vi "Math-NaN Stats.vi"(7 "Array":dbl[](array[numeric])) -> (4 "NaN Mean":dbl, 6 "NaN SD":dbl, 15 "N":i16)   [LabVIEW 2020]
uses:
  <vilib>/Analysis/NI_AALBase.lvlib
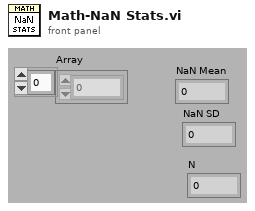
[diagram p1: front panel]
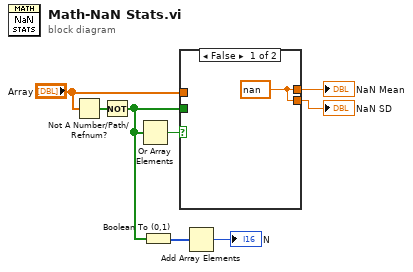
[diagram p0: block diagram]
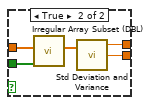
[diagram p2: hidden frame]
diagram:
  n1 = Not A Number/Path/Refnum?(number/path/refnum="Array") -> (NaN/Path/Refnum?=w6:bool[])
  n2 = Not(x=w6) -> (.not. x?=w4:bool[])
  n3 = Or Array Elements(Boolean array=w4) -> (logical OR=w5:bool)
  n4 = Boolean To (0,1)(Boolean=w4) -> (0, 1=w3:i16[])
  n5 = case shown="False" w5 {
    tunnel: [w9 w11] -> w8
    tunnel: "Array" -> [_ w14]
    tunnel: w4 -> [_ w13]
    tunnel: [w9 w10] -> w1
    frame False {
      w9 = nan ("mean")
    }
    frame True {
      n6 = call "Irregular Array Subset (DBL).vi"("Mask"=w13, "Array"=w14) -> ("Array Subset"=w12:dbl[])  [unwired: 8 in, 1 out]
      n7 = call <vilib>:"Std Deviation and Variance.vi"("X"=w12) -> ("mean"=w11:dbl, "standard deviation"=w10:dbl)  [unwired: 1 in, 1 out]
    }
  }
  "NaN Mean" <- w8
  "NaN SD" <- w1
  n8 = Add Array Elements(numeric array=w3) -> (sum=→"N":i16)
